vi "Pause - Resume.vi"(4 "error in (no error)":errorcluster, 5 "Pause/Resume":bool, 6 "Numeric In":i16, 7 "SpeechLib.ISpeechVoice (In)":refnum<k7>) -> (0 "error out":errorcluster, 2 "Numeric Out":i16, 3 "SpeechLib.ISpeechVoice (Out)":refnum<k7>)   [LabVIEW 2018]
doc: "This VI allow you to pause and resume the spoken text. This VI is designed to work in a While loop with one Shift Register wired to the numeric input and output. The case structure contained within this VI is designed to call the pause and the resume commands only once with each press of the same button. The reason for this is due to the way the Microsoft Speech SDK 5.1 software handles the pause and resume commands. The number of resume calls has to equal the number of pause call in order for the speaking of the text to continue. Placing the pause and resume commands in a simple Boolean case structure inside a While Loop would cause the pause and the resume commands to be called multiple times. This would result in delays and other unexpected behavior."
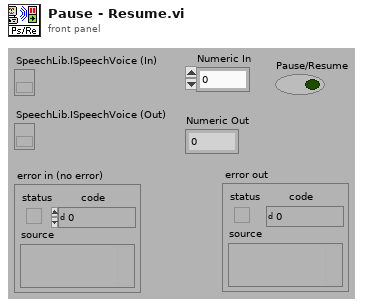
[diagram p1: front panel]
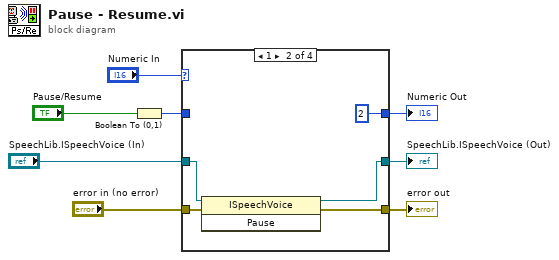
[diagram p0: block diagram]
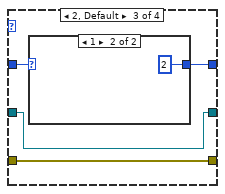
[diagram p3: hidden frame]
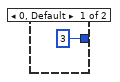
[diagram p4: hidden frame]
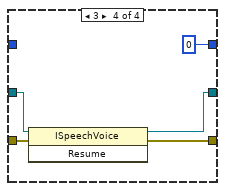
[diagram p5: hidden frame]
diagram:
  n1 = Boolean To (0,1)(Boolean="Pause/Resume") -> (0, 1=w6:i16)
  n2 = case shown="1" "Numeric In" {
    tunnel: [w11 w16 w17 w27] -> w1
    tunnel: [w10 w15 w18 w26] -> w2
    tunnel: "SpeechLib.ISpeechVoice (In)" -> [w11 w14 w17 w25]
    tunnel: "error in (no error)" -> [w10 w13 w18 w24]
    tunnel: w6 -> [w9 _ w20 _]
    tunnel: [w9 i16 2 w19 i16 0] -> w7
    frame 0 {
    }
    frame 1 {
      n3 = invoke class="ISpeechVoice" method="Pause"(reference=w14, error in=w13) -> (reference out=w16:refnum<k7>, error out=w15:errorcluster)  [unwired: 1 in, 1 out]
    }
    frame 2, Default {
      n4 = case shown="1" w20 {
        tunnel: [i16 3 i16 2] -> w19
        frame 0, Default {
        }
        frame 1 {
        }
      }
    }
    frame 3 {
      n5 = invoke class="ISpeechVoice" method="Resume"(reference=w25, error in=w24) -> (reference out=w27:refnum<k7>, error out=w26:errorcluster)  [unwired: 1 in, 1 out]
    }
  }
  "Numeric Out" <- w7
  "error out" <- w2
  "SpeechLib.ISpeechVoice (Out)" <- w1
